vi "Init.vi"(8 "error in (no error)":errorcluster, 11 "Source Name":string) -> (0 "error out":errorcluster, 3 "GetSourceActive out":refnum<class "GetSourceActive.lvclass">)   [LabVIEW 2020, in "obs-websocket.lvlib" / "GetSourceActive.lvclass"]
uses:
  GetSourceActive.lvclass
  GetSourceActive.lvclass/GetSourceActive.ctl
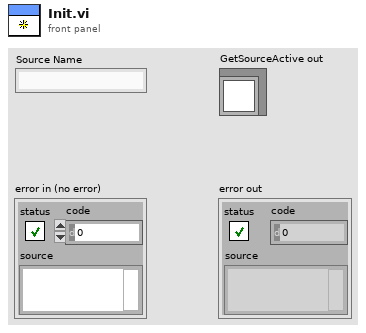
[diagram p1: front panel]
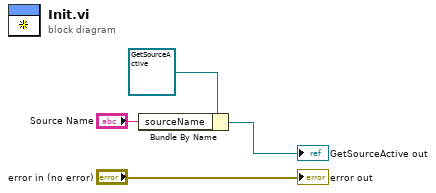
[diagram p0: block diagram]
diagram:
  n1 = Bundle By Name(cluster=refnum<class "GetSourceActive.lvclass"> refnum ("GetSourceActive in"), "sourceName"="Source Name") -> (→"GetSourceActive out":refnum<class "GetSourceActive.lvclass">)
  "error out" <- "error in (no error)"
